vi "CameraReshapeViews.vi"(0 "Cam img in":i16[][](array[numeric]), 1 "XHorizontalSlide":refnum<vi>, 2 "XVerticalSlide":refnum<vi>, 5 "Large Cam ref":refnum<vi>, 7 "Small cam ref":refnum<vi>, 9 "Ions cam ref":refnum<vi>, 11 "error in (no error)":errorcluster, 12 "Large cam coords":T1={"Top :"=1024.0, "Bottom :"=0.0, "Left :"=0.0, "Right :"=1024.0}, 13 "ion coords":T1={"Top :"=107.0, "Bottom :"=100.0, "Left :"=100.0, "Right :"=115.0}) -> (15 "error out":errorcluster)   [LabVIEW 2019]
uses:
  CameraCoordsControl.ctl
  controls/xVerticalSlide/XVerticalSlide.xctl
  controls/xHorizontalSlide/XHorizontalSlide.xctl
  <userlib>/_OpenG.lib/array/array.llb/Reverse 2D Array (I16)__ogtk.vi
panel:
  out "time string":string
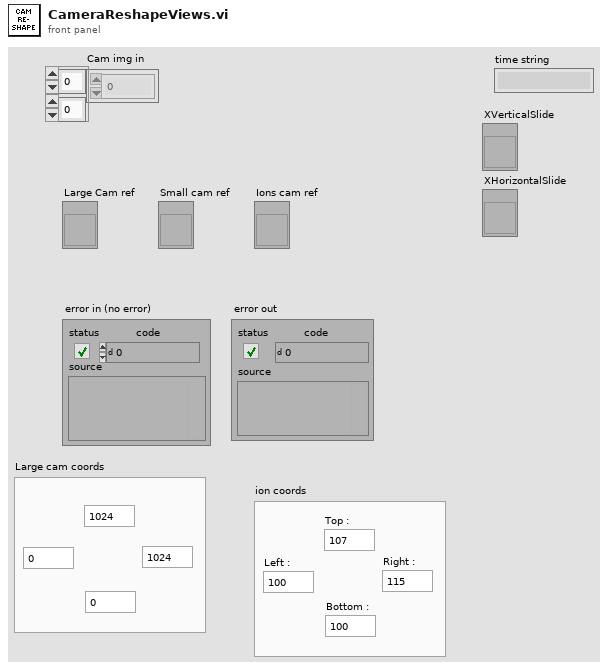
[diagram p1: front panel]
types:
  T1 = typedef "CameraCoordsControl.ctl" = cluster{"Top :":dbl, "Bottom :":dbl, "Left :":dbl, "Right :":dbl}
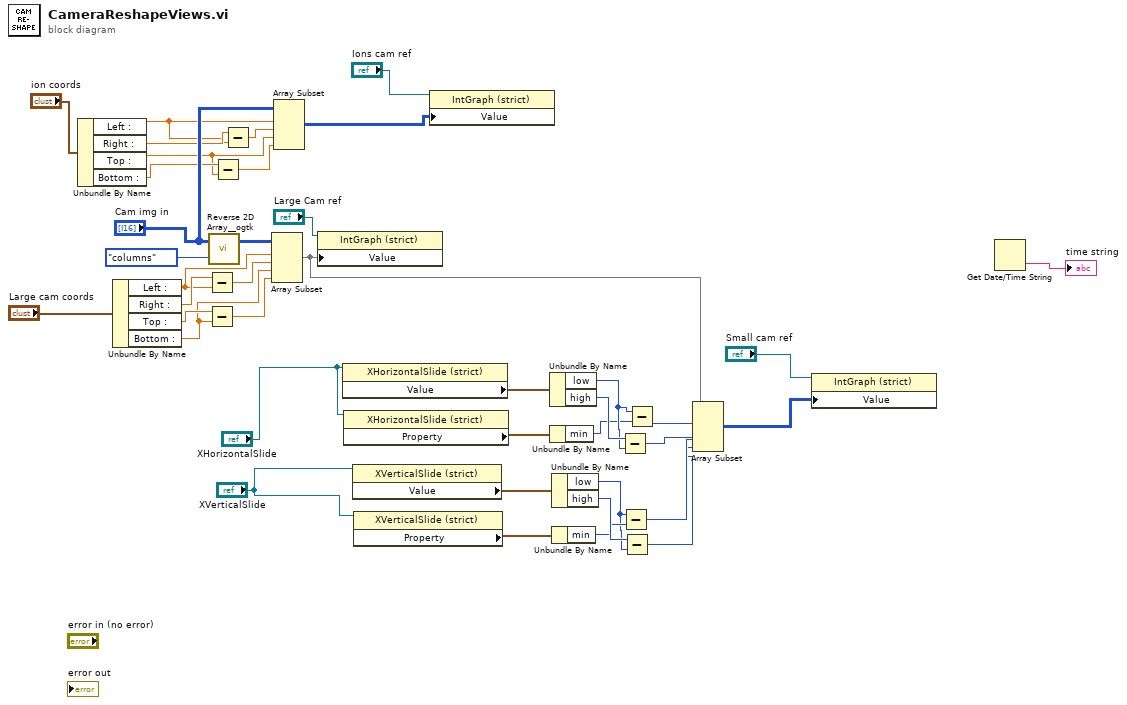
[diagram p0: block diagram]
diagram:
  n1 = Unbundle By Name("ion coords") -> ("Left :"=w5:dbl, "Right :"=w6:dbl, "Top :"=w3:dbl, "Bottom :"=w4:dbl)
  n2 = Unbundle By Name("Large cam coords") -> ("Left :"=w35:dbl, "Right :"=w36:dbl, "Top :"=w32:dbl, "Bottom :"=w31:dbl)
  n3 = Subtract(x=w36, y=w35) -> (x-y=w34:dbl)
  n4 = Subtract(x=w32, y=w31) -> (x-y=w33:dbl)
  n5 = call-poly <userlib>:"Reverse 2D Array__ogtk.vi"("by rows or columns (rows)"=enum16{"rows", "columns"}."columns", "Array"="Cam img in") -> ("Reversed Array"=w38:i16[][])  [unwired: 1 in]
  n6 = Subtract(x=w4, y=w3) -> (x-y=w2:dbl)
  n7 = Subtract(x=w6, y=w5) -> (x-y=w7:dbl)
  n8 = Array Subset(array=w38, index (row)=w35, length (row)=w34, index (col)=w31, length (col)=w33) -> (w29:i16[][])
  n9 = Array Subset(array="Cam img in", index (row)=w5, length (row)=w7, index (col)=w3, length (col)=w2) -> (w10:i16[][])
  n10 = property class="IntGraph (strict)"(reference="Large Cam ref", "Value"=w29) -> ()  [unwired: 1 in, 2 out]
  n11 = property class="XHorizontalSlide (strict)"(reference="XHorizontalSlide") -> ("Value"=w30:cluster{"low":i16, "high":i16})  [unwired: 1 in, 2 out]
  n12 = property class="XHorizontalSlide (strict)"(reference="XHorizontalSlide") -> ("Property"=w27:cluster{"min":i16, "max":i16})  [unwired: 1 in, 2 out]
  n13 = property class="XVerticalSlide (strict)"(reference="XVerticalSlide") -> ("Value"=w23:cluster{"low":i16, "high":i16})  [unwired: 1 in, 2 out]
  n14 = property class="XVerticalSlide (strict)"(reference="XVerticalSlide") -> ("Property"=w22:cluster{"min":i16, "max":i16})  [unwired: 1 in, 2 out]
  n15 = property class="IntGraph (strict)"(reference="Ions cam ref", "Value"=w10) -> ()  [unwired: 1 in, 2 out]
  n16 = Unbundle By Name(w30) -> ("low"=w15:i16, "high"=w25:i16)
  n17 = Unbundle By Name(w27) -> ("min"=w14:i16)
  n18 = Unbundle By Name(w23) -> ("low"=w12:i16, "high"=w21:i16)
  n19 = Unbundle By Name(w22) -> ("min"=w13:i16)
  n20 = Subtract(x=w25, y=w15) -> (x-y=w24:i16)
  n21 = Subtract(x=w12, y=w13) -> (x-y=w19:i16)
  n22 = Subtract(x=w21, y=w12) -> (x-y=w18:i16)
  n23 = Subtract(x=w15, y=w14) -> (x-y=w26:i16)
  n24 = Array Subset(array=w29, index (row)=w26, length (row)=w24, index (col)=w19, length (col)=w18) -> (w17:i16[][])
  n25 = property class="IntGraph (strict)"(reference="Small cam ref", "Value"=w17) -> ()  [unwired: 1 in, 2 out]
  n26 = Get Date/Time String() -> (time string=→"time string":string)  [unwired: 3 in, 1 out]
